vi "IsConnected.vi"(8 "error in (no error)":errorcluster, 11 "TcpReader in":refnum<class "TcpReader.lvclass">) -> (0 "error out":errorcluster, 2 "connected?":bool, 3 "TcpReader out":refnum<class "TcpReader.lvclass">)   [LabVIEW 2025, in "TcpReader.lvclass"]
doc: "Returns TRUE if the Readers connection is alive"
uses:
  TcpReader.lvclass
  TcpReader.lvclass/TcpReader.ctl
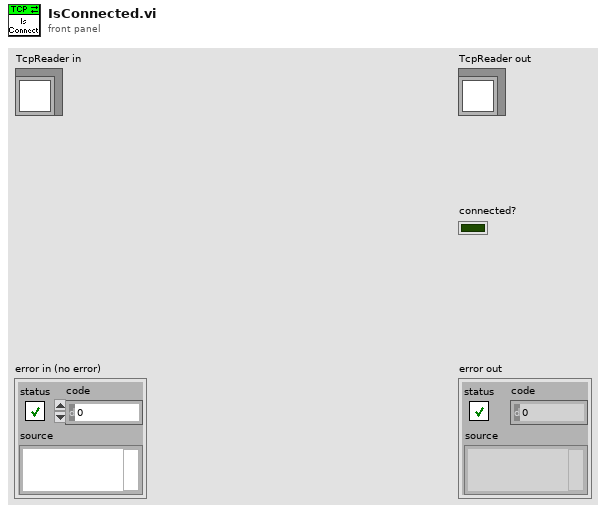
[diagram p1: front panel]
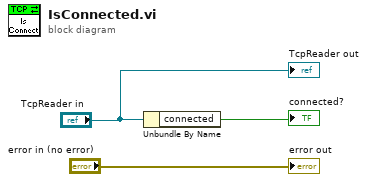
[diagram p0: block diagram]
diagram:
  n1 = Unbundle By Name("TcpReader in") -> ("connected"=→"connected?":bool)
  "error out" <- "error in (no error)"
  "TcpReader out" <- "TcpReader in"
